vi "INTELLIFAUCET Core Start Stop.vi"(7 "mS wait":u32=500, 8 "error in (no error)":errorcluster, 10 "HEWH MW100 Channel Numbers":T1="011", 11 "VISA Refnum in":refnum<visa-resource-name>) -> (0 "error out":errorcluster, 3 "VISA Refnum out":refnum<visa-resource-name>)   [LabVIEW 2016]
uses:
  MW100/Type Definitions/HEWH MW100 Channel Numbers.ctl
  Type Definitions/HEWH Normally Open Valve Control.ctl
panel:
  in  "Tab Control":enum32{"Debug"}(tab)
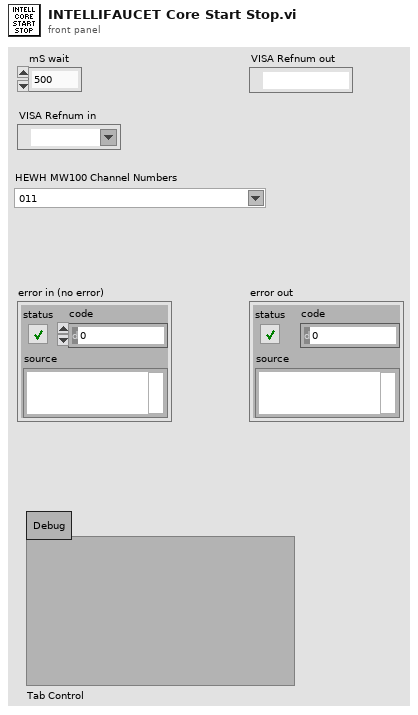
[diagram p1: front panel]
types:
  T1 = typedef "HEWH MW100 Channel Numbers.ctl" = string
  T2 = typedef "HEWH Normally Open Valve Control.ctl" = string
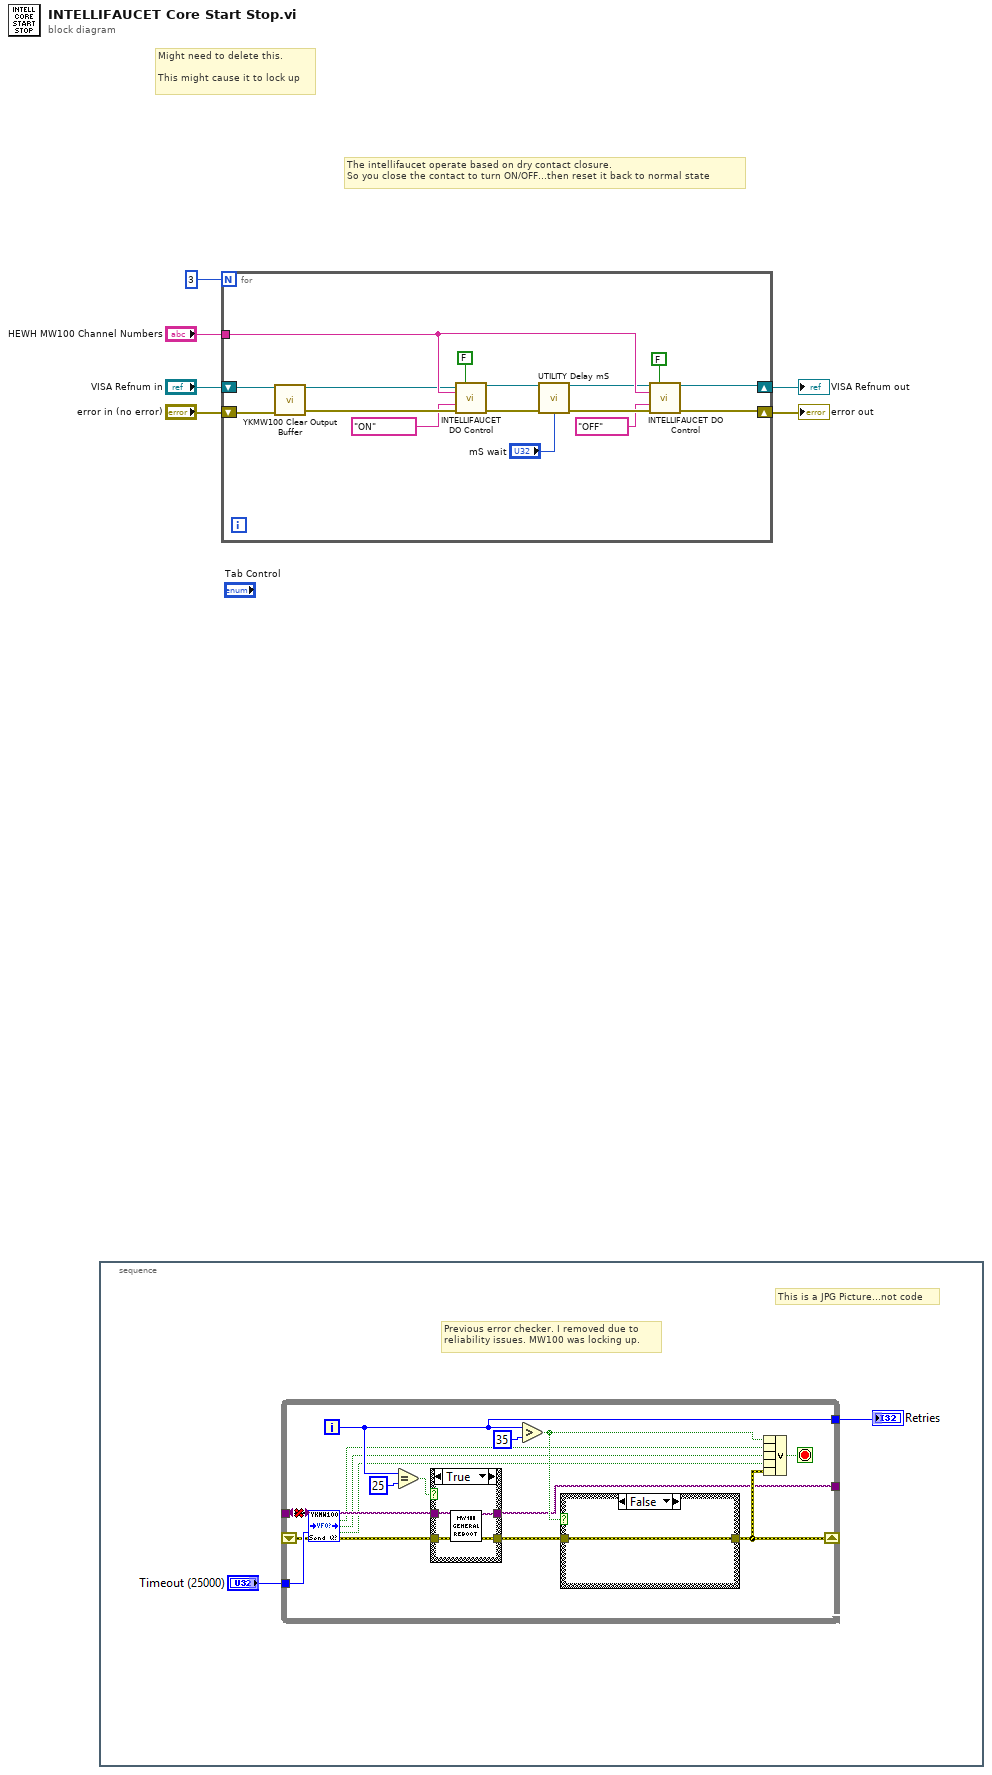
[diagram p0: block diagram]
diagram:
  # "Might need to delete this.\n\nThis might cause it to lock up"
  # "The intellifaucet operate based on dry contact closure. \nSo you close the contact to turn ON/OFF...then reset it back to normal state"
  n1 = stacked-sequence {
    frame #0 {
      # "This is a JPG Picture...not code"
      # "Previous error checker. I removed due to \nreliability issues. MW100 was locking up."
    }
  }
  n2 = for {
    N: 3 -> [_]
    tunnel: "HEWH MW100 Channel Numbers" -> [w17]
    shift-right: [w19] -> w5
    shift-left: "VISA Refnum in" -> [w14]
    shift-right: [w21] -> w6
    shift-left: "error in (no error)" -> [w13]
    n3 = call "YKMW100 Clear Output Buffer.vi"("VISA session"=w14, "error in (no error)"=w13) -> ("dup VISA session"=w15:refnum<visa-resource-name>, "error out"=w16:errorcluster)  [unwired: 12 in]
    n4 = call "INTELLIFAUCET DO Control.vi"("VISA session"=w15, "Normally Closed Valve?"=FALSE, "HEWH MW100 Channel Numbers"=w17, "Normally Open Valve"=T2 "ON", "Error In"=w16) -> ("dup VISA session"=w11:refnum<visa-resource-name>, "error out"=w12:errorcluster)  [unwired: 7 in, 2 out]
    n5 = call "UTILITY Delay mS.vi"("Error In"=w12, "milliseconds to wait"="mS wait") -> ("Error Out"=w20:errorcluster)  [unwired: 13 in]
    n6 = call "INTELLIFAUCET DO Control.vi"("VISA session"=w11, "Normally Closed Valve?"=FALSE, "HEWH MW100 Channel Numbers"=w17, "Normally Open Valve"=T2 "OFF", "Error In"=w20) -> ("dup VISA session"=w19:refnum<visa-resource-name>, "error out"=w21:errorcluster)  [unwired: 7 in, 2 out]
  }
  "error out" <- w6
  "VISA Refnum out" <- w5
